vi "Generate Test Data.vi"(11 "Data in":refnum<class "Data.lvclass">) -> (3 "Data out":refnum<class "Data.lvclass">)   [LabVIEW 2014, in "Base Data Class.lvlib" / "Data.lvclass"]
uses:
  Data.lvclass
  Data.lvclass/Data.ctl
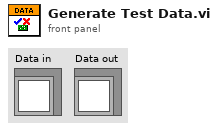
[diagram p1: front panel]
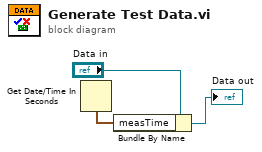
[diagram p0: block diagram]
diagram:
  n1 = Get Date/Time In Seconds() -> (seconds since 1Jan1904=w2:timestamp)
  n2 = Bundle By Name(cluster="Data in", "measTime"=w2) -> (→"Data out":refnum<class "Data.lvclass">)
